vi "Do.vi"(8 "error in":errorcluster, 10 "Actor in":refnum<class "Actor.lvclass">, 11 "Update I16":refnum<class "Update I16.lvclass">) -> (0 "error out":errorcluster, 2 "Actor out":refnum<class "Actor.lvclass">)   [LabVIEW 2014, in "Update I16.lvclass"]
doc: "(<B>Filename</B>: Actor Framework.lvlib:Message.lvclass:Do.vi)\n\nDefines what a message does when it is received by an actor. Generally, a message instructs an actor to invoke one of its methods. By default, this method does nothing. A child class must override it to define behavior. Create a child class by using the Actor Framework Message Maker dialog box."
uses:
  Update I16.lvclass
  <vilib>/ActorFramework/Actor/Actor.lvclass
  Update Setting.lvclass/Update Setting.ctl
  Update I16.lvclass/Update I16.ctl
  <vilib>/NI/Current Value Table/DataTypes/I16_Write.vi
  Read Key.vi
  Read Setting.vi
  <vilib>/NI/Current Value Table/Type to Enum.vi
  <vilib>/NI/Current Value Table/DataTypes/I16_Type To Enum.vi
  <vilib>/NI/Current Value Table/Memory Block.vi
  <vilib>/NI/Current Value Table/DataTypes/I16_Memory Block.vi
  <vilib>/NI/Current Value Table/FGVs/Tag Memory.vi
  <vilib>/NI/Current Value Table/FGVs/CVT Globals.vi
  <vilib>/NI/Current Value Table/Current Value Table.lvlib
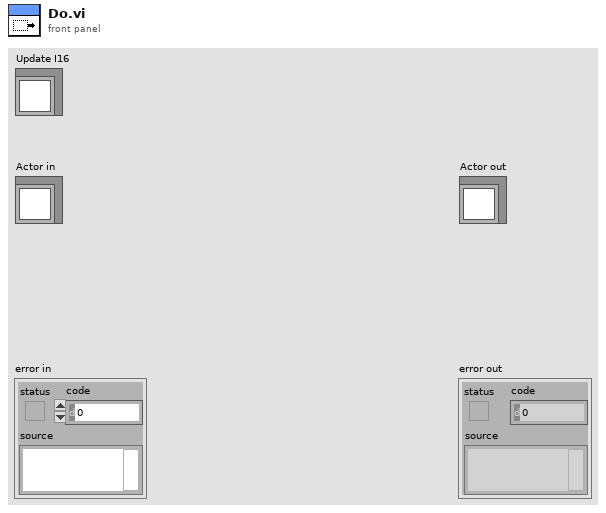
[diagram p1: front panel]
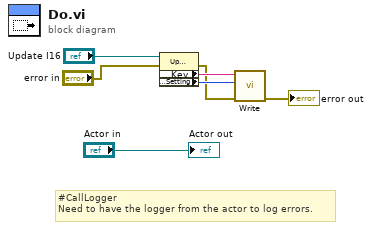
[diagram p0: block diagram]
diagram:
  # "#CallLogger\nNeed to have the logger from the actor to log errors."
  n1 = property class="Update I16.lvclass"(reference="Update I16", error in="error in") -> (error out=w2:errorcluster, "Accessors:Key"=w5:string, "Accessors:Setting"=w4:i16)  [unwired: 1 out]
  n2 = call-poly <vilib>:"Write.vi"("error in (no error)"=w2, "Value"=w4, "Tag Name"=w5) -> ("error out"=→"error out":errorcluster)  [unwired: 8 in]
  "Actor out" <- "Actor in"
